vi "rqcBob Configure PD use window.vi"(8 "error in":errorcluster, 10 "PD.use window":bool, 11 "FPGA reference in":refnum<k20>) -> (0 "error out":errorcluster, 3 "FPGA reference out":refnum<k20>)   [LabVIEW 2018]
uses:
  <vilib>/Utility/error.llb/Error Cluster From Error Code.vi
  <vilib>/rvi/errors/niLvFpgaAdjustHostInterfaceError.vi
  <vilib>/rvi/interface/nirviReadWriteControl/nirviReadWriteControl.xnode
  NiFpgaLv.dll
  <vilib>/rvi/interface/Simulation/niFpgaSimulationCallBeginRW.vi
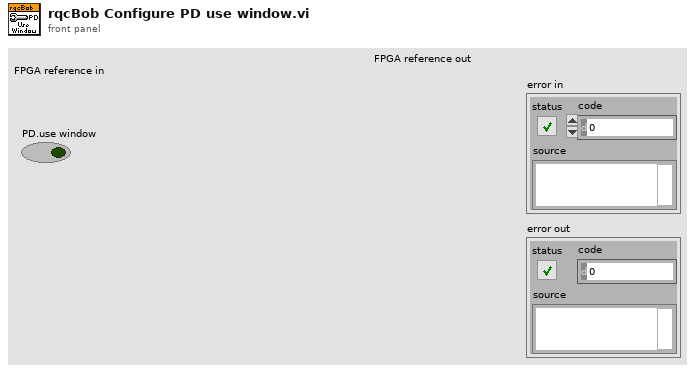
[diagram p1: front panel]
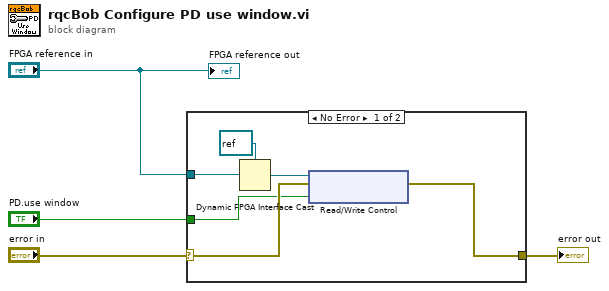
[diagram p0: block diagram]
diagram:
  n1 = case shown="No Error" "error in" {
    selector: "error in" -> [w10 w11]
    tunnel: [w9 w11] -> w2
    tunnel: "FPGA reference in" -> [w7 _]
    tunnel: "PD.use window" -> [w5 _]
    frame No Error {
      n2 = Dynamic FPGA Interface Cast(Session In=refnum<k20> refnum ("FPGA Interface"), Type=w7) -> (Session Out=w6:refnum<k20>)
      n3 = xnode "Read/Write Control"("FPGA VI Reference In"=w6, "error in"=w10, "PD.use window"=w5) -> ("error out"=w9:errorcluster)  [unwired: 1 out]
    }
    frame Error {
    }
  }
  "error out" <- w2
  "FPGA reference out" <- "FPGA reference in"
